vi "Autonomous Independent.vi"   [LabVIEW 2014]
doc: "This VI is called when autonomous begins, and will automatically be terminated when autonomous ends. You can carry out timed or sensor driven robot movement independently without needing to return to the caller."
uses:
  <vilib>/Rock Robotics/WPI/Solenoid/WPI_SolenoidValue.ctl
  <vilib>/Rock Robotics/WPI/Joystick/WPI_JoystickGetSetRefNum.vi
  <vilib>/Rock Robotics/WPI/RobotDrive/WPI_RobotDriveGetSetRefNum.vi
  <vilib>/Rock Robotics/WPI/Solenoid/WPI_SolenoidSetEnum.vi
  <vilib>/Rock Robotics/WPI/RobotDrive/WPI_RobotDriveArcadeDrive_Standard(NoSaturation).vi
panel:
  # "Be sure to right-click and choose Data Operations>>Make Current Value default if you want to save the array values with the VI"
types:
  T1 = typedef "WPI_JoystickDevRef.ctl" = cluster{"Device":T2}
  T2 = typedef "WPI_JoystickDeviceEnum.ctl" = enum16{"USB 0", "USB 1", "USB 2", "USB 3", "USB 4", "USB 5"}
  T3 = typedef "WPI_RobotDriveDevRef.ctl" = cluster{"DevStatus":errorcluster, "Motors[]":T4[], "Square Inputs":bool, "Max Output":dbl}
  T4 = typedef "WPI_MotorControlDeviceRef.ctl" = cluster{"DeviceStatus":errorcluster, "Type":T5, "PWM":cluster{"Controller":T6, "PWM Channel":T7, "DeadBand":T8}, "CAN":cluster{"Device Number":u8, "Control Mode":T9, "Semaphore":T10, "Max Vout":dbl, "TalonSRX Control Mode":T11}, "Invert":bool, "TransformRef":T12, "InvTransformRef":T12}
  T5 = typedef "WPI_MotorControlType.ctl" = enum16{"PWM", "CAN", "CANTalonSRX"}
  T6 = typedef "FPGA_TypedefDigitalModule.ctl" = enum16{"Controller 1"}
  T7 = typedef "FPGA_DIOPWMChannel.ctl" = enum8{"PWM 0", "PWM 1", "PWM 2", "PWM 3", "PWM 4", "PWM 5", "PWM 6", "PWM 7", "PWM 8", "PWM 9", "PWM MXP 0", "PWM MXP 1", "PWM MXP 2", "PWM MXP 3", "PWM MXP 4", "PWM MXP 5", "PWM MXP 6", "PWM MXP 7", "PWM MXP 8", "PWM MXP 9", "Invalid"}
  T8 = typedef "WPI_PWMDeadband.ctl" = cluster{"Name":string, "maxPositivePwm":i32, "minPositivePwm":i32, "centerPwm":i32, "maxNegativePwm":i32, "minNegativePwm":i32, "angularRange":u16}
  T9 = typedef "WPI_CANJaguar_ControlMode.ctl" = enum8{"Percent VBus", "Current", "Speed", "Position", "Voltage"}
  T10 = typedef "Semaphore RefNum" = refnum<k1>
  T11 = typedef "WPI_CANTalonSRX_APIControlMode.ctl" = enum8{"Percent VBus", "Speed", "Position", "Slave", "Unchanged / Invalid"}
  T12 = typedef "WPI_PWMTransform_ConPane.ctl" = refnum<vi>
  T13 = typedef "WPI_SolenoidDevRef.ctl" = cluster{"DevStatus":errorcluster, "Pneumatics Control Module":u8, "Forward Solenoid Channel":T14, "Reverse Solenoid Channel":T14}
  T14 = typedef "WPI_SolenoidChannel.ctl" = enum8{"Solenoid 0", "Solenoid 1", "Solenoid 2", "Solenoid 3", "Solenoid 4", "Solenoid 5", "Solenoid 6", "Solenoid 7", "Invalid"}
  T15 = typedef "WPI_SolenoidValue.ctl" = enum16{"Off", "On", "Forward", "Reverse"}
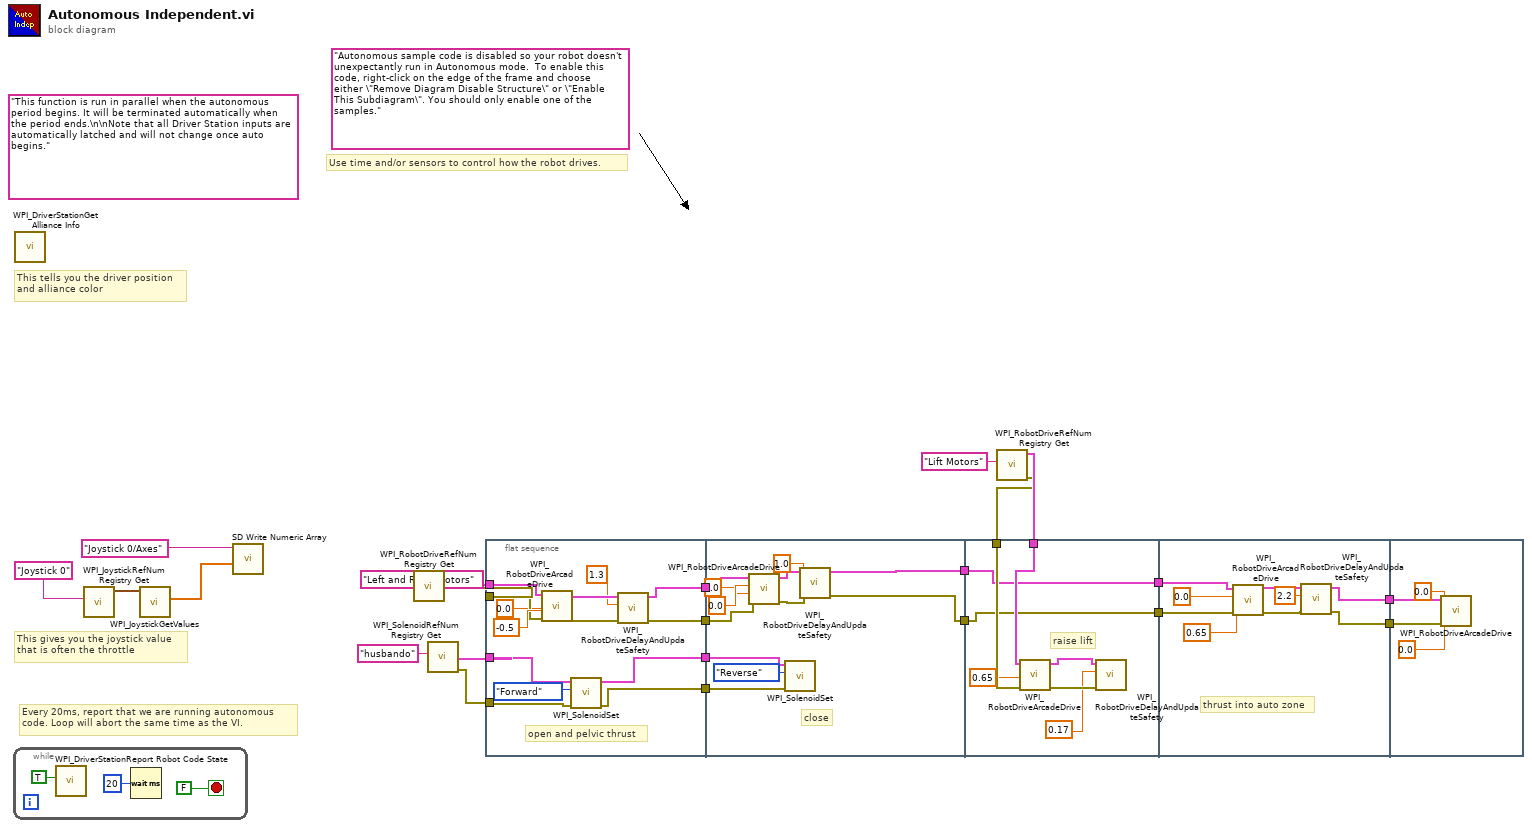
[diagram p0: block diagram]
diagram:
  (unwired) "Autonomous sample code is disabled so your robot doesn't unexpectantly run in Autonomous mode.  To enable this code, right-click on the edge of the frame and choose either \"Remove Diagram Disable Structure\" or \"Enable This Subdiagram\". You should only enable one of the samples."
  (unwired) "This function is run in parallel when the autonomous period begins. It will be terminated automatically when the period ends.\n\nNote that all Driver Station inputs are automatically latched and will not change once auto begins."
  # "Every 20ms, report that we are running autonomous\ncode. Loop will abort the same time as the VI."
  # "This gives you the joystick value\nthat is often the throttle"
  # "Use time and/or sensors to control how the robot drives."
  # "This tells you the driver position\nand alliance color"
  n1 = while {
    stop <- FALSE stop-if-true
    n2 = call <vilib>:"WPI_DriverStationReport Robot Code State.vi"("Autonomous"=TRUE) -> ()  [unwired: 10 in, 1 out]
    n3 = Wait (ms)(milliseconds to wait=u32 20) -> ()  [unwired: 1 out]
  }
  n4 = call <vilib>:"WPI_DriverStationGet Alliance Info.vi"() -> ()  [unwired: 12 out]
  n5 = call <vilib>:"WPI_JoystickRefNum Registry Get.vi"("refnum name"="Joystick 0") -> ("JoystickDevRef"=w22:T1)  [unwired: 1 in, 9 out]
  n6 = call <vilib>:"WPI_JoystickGetValues.vi"("JoystickDevRef"=w22) -> ("Axes"=w20:dbl[])  [unwired: 6 in, 4 out]
  n7 = call <vilib>:"SD Write Numeric Array.vi"("Numeric Array"=w20, "Name"="Joystick 0/Axes") -> ()  [unwired: 8 in, 2 out]
  n8 = call <vilib>:"WPI_RobotDriveRefNum Registry Get.vi"("refnum name"="Left and Right Motors") -> ("error out"=w16:errorcluster, "RobotDriveDevRef"=w17:T3)  [unwired: 9 in]
  n9 = call <vilib>:"WPI_SolenoidRefNum Registry Get.vi"("refnum name"="husbando") -> ("error out"=w10:errorcluster, "SolenoidDevRef"=w15:T13)  [unwired: 9 in]
  n10 = flat-sequence {
    tunnel: w17 -> [w40]
    tunnel: w16 -> [w36]
    tunnel: w15 -> [w33]
    tunnel: [w32] -> w14
    tunnel: [w30] -> w13
    tunnel: [w29] -> w12
    tunnel: [w28] -> w11
    tunnel: w10 -> [w27]
    tunnel: w14 -> [w47]
    tunnel: w13 -> [w52]
    tunnel: w12 -> [w46]
    tunnel: w11 -> [w50]
    tunnel: [w43] -> w9
    tunnel: [w42] -> w8
    tunnel: w9 -> [w53]
    tunnel: w8 -> [w54]
    tunnel: w6 -> [w60]
    tunnel: w5 -> [w59]
    tunnel: [w54] -> w2
    tunnel: [w53] -> w1
    tunnel: [w64] -> w4
    tunnel: [w63] -> w3
    tunnel: w2 -> [w62]
    tunnel: w1 -> [w61]
    tunnel: w4 -> [w73]
    tunnel: w3 -> [w72]
    frame #0 {
      # "open and pelvic thrust"
      n11 = call-poly <vilib>:"WPI_RobotDriveArcadeDrive.vi"("error in (no error)"=w36, "Y axis value"=-0.5, "X axis value"=0.0, "RobotDriveDevRef"=w40) -> ("error out"=w37:errorcluster, "RobotDriveDevRef"=w38:T3)  [unwired: 5 in, 1 out]
      n12 = call-poly <vilib>:"WPI_SolenoidSet.vi"("error in (no error)"=w27, "Value"=WPI_SolenoidValue."Forward", "SolenoidDevRef"=w33) -> ("error out"=w28:errorcluster, "SolenoidDevRef"=w30:T13)  [unwired: 7 in]
      n13 = call <vilib>:"WPI_RobotDriveDelayAndUpdateSafety.vi"("error in (no error)"=w37, "Delay (s)"=1.3, "RobotDriveDevRef"=w38) -> ("error out"=w29:errorcluster, "RobotDriveDevRef 2"=w32:T3)  [unwired: 7 in]
    }
    frame #1 {
      # "close"
      n14 = call-poly <vilib>:"WPI_RobotDriveArcadeDrive.vi"("error in (no error)"=w46, "Y axis value"=0.0, "X axis value"=0.0, "RobotDriveDevRef"=w47) -> ("error out"=w45:errorcluster, "RobotDriveDevRef"=w44:T3)  [unwired: 5 in, 1 out]
      n15 = call-poly <vilib>:"WPI_SolenoidSet.vi"("error in (no error)"=w50, "Value"=WPI_SolenoidValue."Reverse", "SolenoidDevRef"=w52) -> ()  [unwired: 7 in, 2 out]
      n16 = call <vilib>:"WPI_RobotDriveDelayAndUpdateSafety.vi"("error in (no error)"=w45, "Delay (s)"=1.0, "RobotDriveDevRef"=w44) -> ("error out"=w43:errorcluster, "RobotDriveDevRef 2"=w42:T3)  [unwired: 7 in]
    }
    frame #2 {
      # "raise lift"
      n17 = call-poly <vilib>:"WPI_RobotDriveArcadeDrive.vi"("error in (no error)"=w59, "Y axis value"=0.65, "RobotDriveDevRef"=w60) -> ("error out"=w56:errorcluster, "RobotDriveDevRef"=w57:T3)  [unwired: 6 in, 1 out]
      n18 = call <vilib>:"WPI_RobotDriveDelayAndUpdateSafety.vi"("error in (no error)"=w56, "Delay (s)"=0.17, "RobotDriveDevRef"=w57) -> ()  [unwired: 7 in, 2 out]
    }
    frame #3 {
      # "thrust into auto zone"
      n19 = call-poly <vilib>:"WPI_RobotDriveArcadeDrive.vi"("error in (no error)"=w61, "Y axis value"=0.65, "X axis value"=0.0, "RobotDriveDevRef"=w62) -> ("error out"=w66:errorcluster, "RobotDriveDevRef"=w67:T3)  [unwired: 5 in, 1 out]
      n20 = call <vilib>:"WPI_RobotDriveDelayAndUpdateSafety.vi"("error in (no error)"=w66, "Delay (s)"=2.2, "RobotDriveDevRef"=w67) -> ("error out"=w63:errorcluster, "RobotDriveDevRef 2"=w64:T3)  [unwired: 7 in]
    }
    frame #4 {
      n21 = call-poly <vilib>:"WPI_RobotDriveArcadeDrive.vi"("error in (no error)"=w72, "Y axis value"=0.0, "X axis value"=0.0, "RobotDriveDevRef"=w73) -> ()  [unwired: 5 in, 3 out]
    }
  }
  n22 = call <vilib>:"WPI_RobotDriveRefNum Registry Get.vi"("refnum name"="Lift Motors") -> ("error out"=w5:errorcluster, "RobotDriveDevRef"=w6:T3)  [unwired: 9 in]
